vi "SR830 set frequency.vi"(8 "error in (no error)":errorcluster, 10 "frequency":dbl[unit], 11 "VISA resource name":refnum<visa-resource-name>) -> (0 "error out":errorcluster, 3 "VISA resource name out":refnum<visa-resource-name>)   [LabVIEW 2009, in "SR830.lvlib"]
doc: "Sets the current frequency of the lock-in amplifier. Note: to set the frequency, the lock-in reference mode must first be set to internal."
uses:
  SR830.lvlib
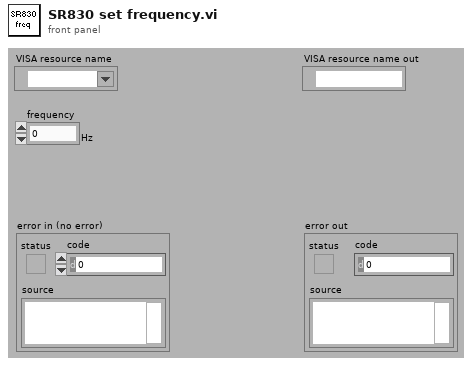
[diagram p1: front panel]
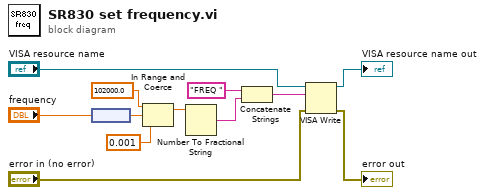
[diagram p0: block diagram]
diagram:
  n1 = node("frequency") -> (w1:dbl)
  n2 = In Range and Coerce(upper limit=102000.0, x=w1, lower limit=0.001) -> (coerced(x)=w12:dbl)  [unwired: 1 out]
  n3 = Number To Fractional String(number=w12) -> (F-format string=w9:string)  [unwired: 3 out]
  n4 = Concatenate Strings("FREQ " ("write buffer"), w9) -> (w4:string)
  n5 = VISA Write(VISA resource name="VISA resource name", write buffer=w4, error in (no error)="error in (no error)") -> (VISA resource name out=→"VISA resource name out":refnum<visa-resource-name>, error out=→"error out":errorcluster)  [unwired: 1 out]
